vi "NET_Rotation.vi"(8 "Read(F) Write(T)":bool, 11 "Offset In":dbl) -> (3 "Offset Out":dbl)   [LabVIEW 2017]
uses:
  <vilib>/Rock Robotics/Network Tables/NT Read Number.vi
  <vilib>/Rock Robotics/Network Tables/NT Write Number.vi
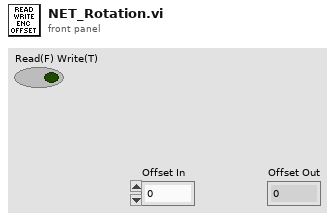
[diagram p1: front panel]
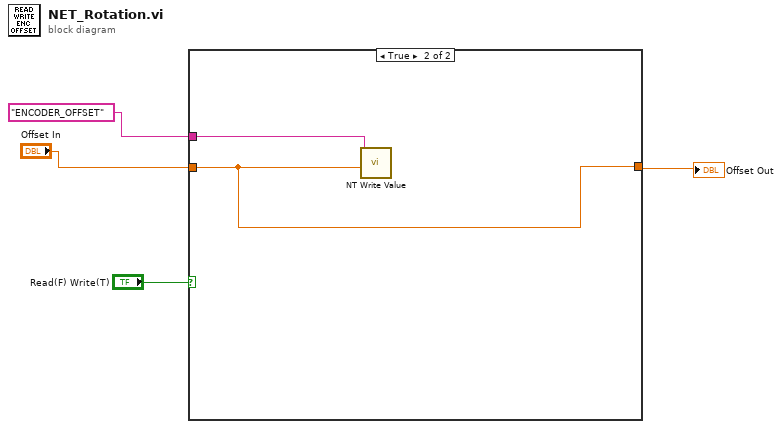
[diagram p0: block diagram]
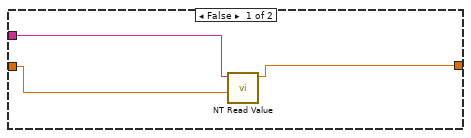
[diagram p2: hidden frame]
diagram:
  n1 = case shown="True" "Read(F) Write(T)" {
    tunnel: "ENCODER_OFFSET" ("Name") -> [w7 w9]
    tunnel: "Offset In" -> [w6 w8]
    tunnel: [w5 w8] -> w2
    frame False {
      n2 = call-poly <vilib>:"NT Read Value.vi"("Default Value"=w6, "Name"=w7) -> ("Numeric"=w5:dbl)  [unwired: 8 in, 1 out]
    }
    frame True {
      n3 = call-poly <vilib>:"NT Write Value.vi"("Numeric"=w8, "Name"=w9) -> ()  [unwired: 9 in, 1 out]
    }
  }
  "Offset Out" <- w2
